vi "Create Instrument Addon.vi"(8 "Error In":errorcluster, 9 "PCL Decimation":u16, 10 "Protocol In":refnum<class "Protocol Parent.lvclass">, 11 "Target in":refnum<k24>) -> (0 "Error Out":errorcluster, 2 "Instrument Addon Refnum Out":T1=18446744073709551615 format="%.0x", 3 "Target Out":refnum<k24>)   [LabVIEW 2018, in "Instrument Addon Scripting API.lvlib"]
uses:
  Instrument Addon Scripting API.lvlib
  NationalInstruments.VeriStand.SystemDefinitionAPI
  Addon/Support Libraries/Protocols.lvlibp/Protocol Parent/Protocol Parent.lvclass
  <vilib>/NI Veristand/Custom Device API/Custom Device Item Ref.ctl
  <vilib>/NI Veristand/Custom Device API/Custom Device API.lvlib
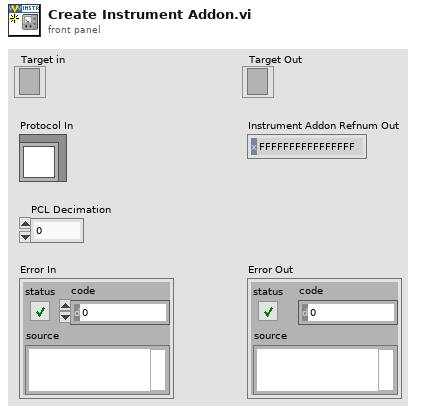
[diagram p1: front panel]
types:
  T1 = typedef "Custom Device API.lvlib/Custom Device Item Ref.ctl" = u64
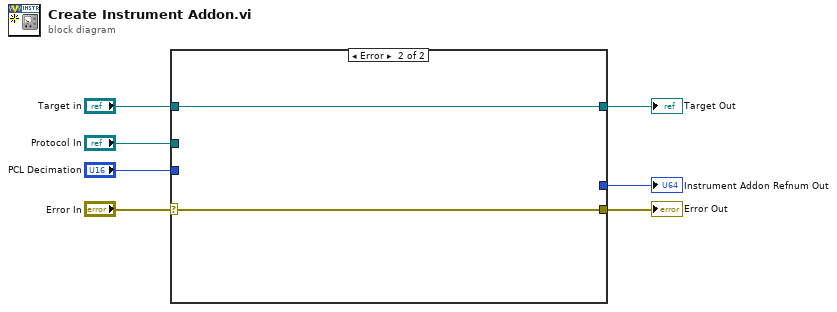
[diagram p0: block diagram]
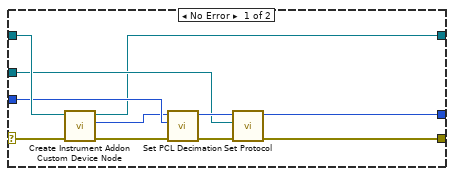
[diagram p2: hidden frame]
diagram:
  n1 = case shown="Error" "Error In" {
    selector: "Error In" -> [w18 w19]
    tunnel: "Target in" -> [w17 w20]
    tunnel: "Protocol In" -> [w11 _]
    tunnel: "PCL Decimation" -> [w15 _]
    tunnel: [w10 w20] -> w3
    tunnel: [w9 _] -> w2
    tunnel: [w8 w19] -> w1
    frame No Error {
      n2 = call "Create Instrument Addon Custom Device Node.vi"("Error In"=w18, "Target In"=w17) -> ("Error Out"=w16:errorcluster, "Instrument Addon Refnum Out"=w14:u64, "Target Out"=w10:refnum<k24>)  [unwired: 7 in]
      n3 = call "Set PCL Decimation.vi"("Error In"=w16, "PCL Decimation"=w15, "Instrument Addon Refnum In"=w14) -> ("Error Out"=w13:errorcluster, "Instrument Addon Refnum Out"=w12:T1)  [unwired: 7 in]
      n4 = call "Set Protocol.vi"("Error In"=w13, "Protocol in"=w11, "Instrument Addon Refnum In"=w12) -> ("Error Out"=w8:errorcluster, "Instrument Addon Refnum Out"=w9:T1)  [unwired: 7 in]
    }
    frame Error {
    }
  }
  "Target Out" <- w3
  "Instrument Addon Refnum Out" <- w2
  "Error Out" <- w1
